vi "Inject Attribute List.vi"(6 "Attributes Ref":refnum<data-value>, 8 "error in (no error)":errorcluster, 11 "Stop Under Body Wash in":refnum<class "Stop Under Body Wash.lvclass">) -> (0 "error out":errorcluster, 3 "Stop Under Body Wash out":refnum<class "Stop Under Body Wash.lvclass">)   [LabVIEW 2019, in "Stop Under Body Wash.lvclass"]
uses:
  <vilib>/gpm_packages/@cs/Car-wash/Source/Process Steps/Stop Under Body Wash/Stop Under Body Wash.lvclass
  <vilib>/gpm_packages/@cs/lookup-table/Source/LookupTable/LookupTable.lvclass
  <vilib>/gpm_packages/@cs/lookup-table/Source/LookupTable/LookupTable.lvclass/LookupTable.ctl
  <vilib>/gpm_packages/@cs/Car-wash/Source/Process Steps/Stop Under Body Wash/Stop Under Body Wash.lvclass/Stop Under Body Wash.ctl
  ab4fc44f-7cf6-45f7-a1fd-3880feaf2b28.vi
  <vilib>/gpm_packages/@cs/lookup-table/Source/LookupTable/Read Table Reference.vi
  ab4fc44f-7cf6-45f7-a1fd-3880feaf2b28.vi/a111f7e7-8271-4895-8f24-758ffde8e811.vi
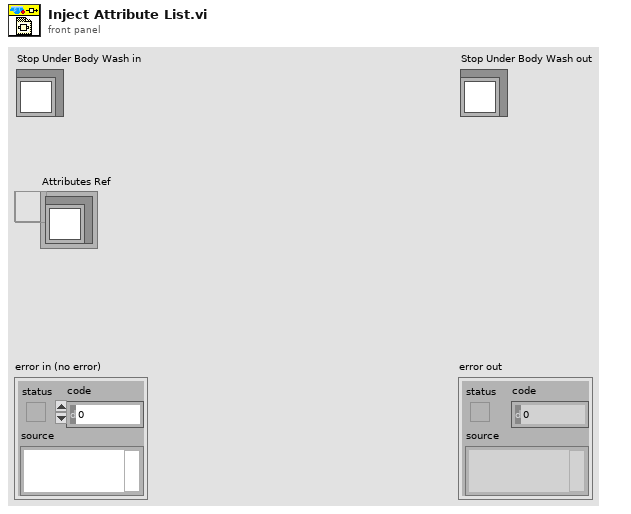
[diagram p1: front panel]
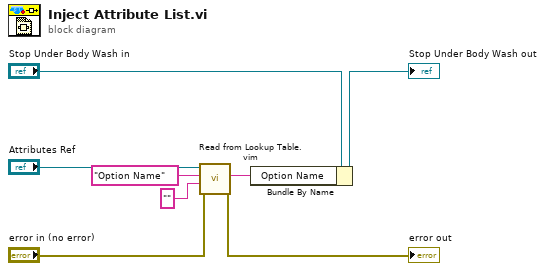
[diagram p0: block diagram]
diagram:
  n1 = call "Read from Lookup Table.vim"("error in (no error)"="error in (no error)", "Type"="", "Item Name"="Option Name", "LookupTable Reference"="Attributes Ref") -> ("error out"=→"error out":errorcluster, "Value"=w6:string)  [unwired: 4 in, 2 out]
  n2 = Bundle By Name(cluster="Stop Under Body Wash in", "Option Name"=w6) -> (→"Stop Under Body Wash out":refnum<class "Stop Under Body Wash.lvclass">)
